vi "MQTT Connect.vi"(8 "error in (no error)":errorcluster, 10 "Username/Password":string, 11 "Secured TCP Connection":refnum<class "Connection.TCP-TLS.lvclass">) -> (0 "error out":errorcluster, 2 "connected":bool, 3 "Client out":refnum<class "Client.lvclass">)   [LabVIEW 2021]
uses:
  <vilib>/LabVIEW Open Source Project/MQTT Client/Client class/Client.lvclass
  C:/Program Files (x86)/National Instruments/LabVIEW 2021/vi.lib/LabVIEW Open Source Project/MQTT Connection/MQTT_Base/Base Class/MQTT_Base.lvclass
  <vilib>/LabVIEW Open Source Project/MQTT Secured TCP Connection/Connection.SecuredTCP/Connection.TCP-TLS.lvclass
  C:/Program Files (x86)/National Instruments/LabVIEW 2021/vi.lib/LabVIEW Open Source Project/Connection/Connection/Connection.lvclass
  <vilib>/LabVIEW Open Source Project/MQTT Control Packets/Control Packets/CONNECT/ConnectFlags -- cluster.ctl
  <vilib>/LabVIEW Open Source Project/MQTT Client/Client class/Client.lvclass/Client.ctl
  <vilib>/LabVIEW Open Source Project/MQTT Connection/MQTT_Base/Base Class/MQTT_Base.lvclass/MQTT_Base.ctl
  <vilib>/LabVIEW Open Source Project/MQTT Control Packets/Control Packets/PUBLISH/PUBLISH.lvclass
  <vilib>/LabVIEW Open Source Project/MQTT Connection/MQTT_Base/Base Class/MQTT_Base.lvclass
  <vilib>/LabVIEW Open Source Project/MQTT Control Packets/Control Packets/CONNECT/CONNECT.lvclass
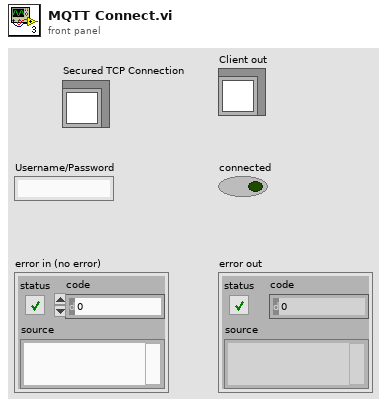
[diagram p1: front panel]
types:
  T1 = typedef "MQTT_Control_Packets.lvlib/CONNECT.lvclass/ConnectFlags -- cluster.ctl" = cluster{"Reserved":bool, "Clean Session":bool, "Will Flag":bool, "Will QoS 1":bool, "Will QoS 2":bool, "Will Retain":bool, "Password Flag":bool, "User Name Flag":bool}
  T2 = cluster{"Will Topic":string, "Will Message":string, "Username":string, "Password":string}
  T3 = typedef "MQTT Client.lvlib/Client.lvclass/Public Events -- cluster.ctl" = cluster{"Connection Status":refnum<user-event>, "Connected":refnum<user-event>, "Application Message":refnum<user-event>}
  T4 = typedef "MQTT Base.lvlib/MQTT_Base.lvclass/Public Events -- cluster.ctl" = cluster{"Stop Event":refnum<user-event>, "Error Event":refnum<user-event>, "Inbound Message":refnum<user-event>}
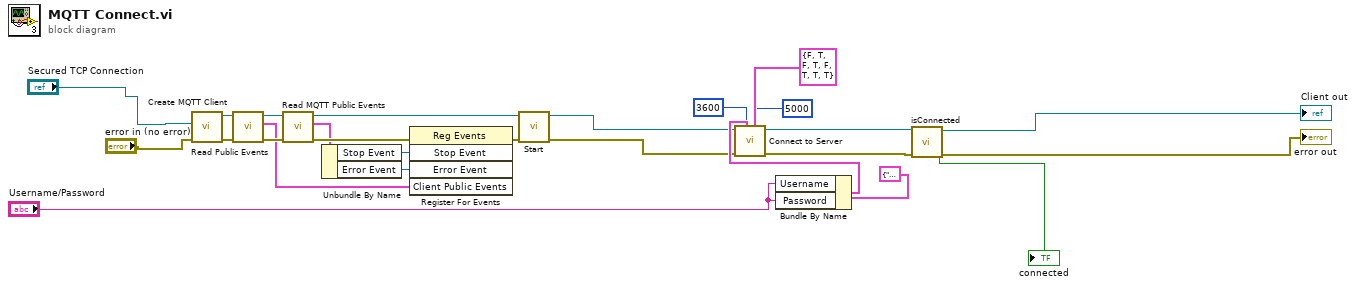
[diagram p0: block diagram]
diagram:
  n1 = call <vilib>:"Create MQTT Client.vi"("error in (no error)"="error in (no error)", "Connection Configuration"="Secured TCP Connection") -> ("error out"=w12:errorcluster, "Client out"=w14:refnum<class "Client.lvclass">)  [unwired: 8 in]
  n2 = call <vilib>:"Read Public Events.vi"("error in (no error)"=w12, "Client in"=w14) -> ("error out"=w11:errorcluster, "Client Public Events"=w9:T3, "Client out"=w13:refnum<class "Client.lvclass">)  [unwired: 7 in]
  n3 = call <vilib>:"Read MQTT Public Events.vi"("error in (no error)"=w11, "MQTT_Base in"=w13) -> ("error out"=w10:errorcluster, "MQTT Public Events"=w4:T4, "MQTT_Base out"=w7:refnum<class "Client.lvclass">)  [unwired: 7 in]
  n4 = Unbundle By Name(w4) -> ("Stop Event"=w6:refnum<user-event>, "Error Event"=w5:refnum<user-event>)
  n5 = register-events(error in=w10, w6, w5, w9) -> (error out=w8:errorcluster)  [unwired: 1 in, 1 out]
  n6 = call <vilib>:"Start.vi"("error in (no error)"=w8, "MQTT_Base in"=w7) -> ("error out"=w2:errorcluster, "MQTT_Base out"=w3:refnum<class "Client.lvclass">)  [unwired: 7 in, 1 out]
  n7 = Bundle By Name(cluster=T2 {"Will Topic"="", "Will Message"="", "Username"="", "Password"=""} ("Payload"), "Username"="Username/Password", "Password"="Username/Password") -> (w24:T2)
  n8 = call <vilib>:"Connect to Server.vi"("timeout (2000 ms)"=5000, "Connect Flags"=T1 {"Reserved"=FALSE, "Clean Session"=TRUE, "Will Flag"=FALSE, "Will QoS 1"=TRUE, "Will QoS 2"=FALSE, "Will Retain"=TRUE, "Password Flag"=TRUE, "User Name Flag"=TRUE}, "Keep Alive (s)"=u16 3600, "Payload"=w24, "error in (no error)"=w2, "Client in"=w3) -> ("error out"=w19:errorcluster, "Client out"=w20:refnum<class "Client.lvclass">)  [unwired: 2 in, 2 out]
  n9 = call <vilib>:"isConnected.vi"("error in (no error)"=w19, "Client in"=w20) -> ("error out"=→"error out":errorcluster, "connected"=→"connected":bool, "Client out"=→"Client out":refnum<class "Client.lvclass">)  [unwired: 7 in]
